vi "MaxAndMin.vi"() -> ()   [LabVIEW 2018]
panel:
  out "error out":errorcluster
  in  "Numbers":dbl[](array[numeric])=[0.0, -345.0, 245352.0, 23.0]
  out "Max and Min":cluster{"Max":dbl, "Min":dbl}
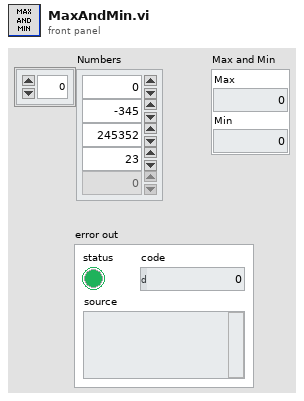
[diagram p1: front panel]
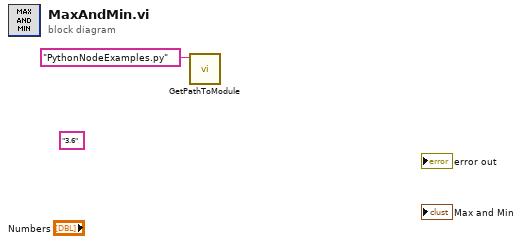
[diagram p0: block diagram]
diagram:
  (unwired) "3.6" ("Python version")
  n1 = call "GetPathToModule.vi"("module name"="PythonNodeExamples.py") -> ()  [unwired: 10 in, 1 out]
